vi "Output_Trav_Pos.vi"(4 "Positions to Output":T1) -> (1 "error out":errorcluster)   [LabVIEW 2011]
uses:
  Controls/Positions.ctl
  Globals/Trav_pos_global.vi
  <userlib>/LV-Link3/PolySubVIs/DtCreateAoutChan.vi
  Route mapping/Route_mapping_global.vi
  <userlib>/LV-Link3/PolySubVIs/DtOLWriteSingle.vi
  <userlib>/LV-Link3/PolySubVIs/DtOLWriteMultiple2D.vi
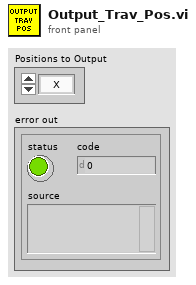
[diagram p1: front panel]
types:
  T1 = typedef "Positions.ctl" = enum16{"X", "Y", "Z", "XY", "XZ", "YZ", "XYZ"}
  T2 = typedef "Box_size.ctl" = cluster{"Max":dbl, "Min":dbl}[]
  T3 = enum32{"Bad", "Idle", "Run top level", "Running"}
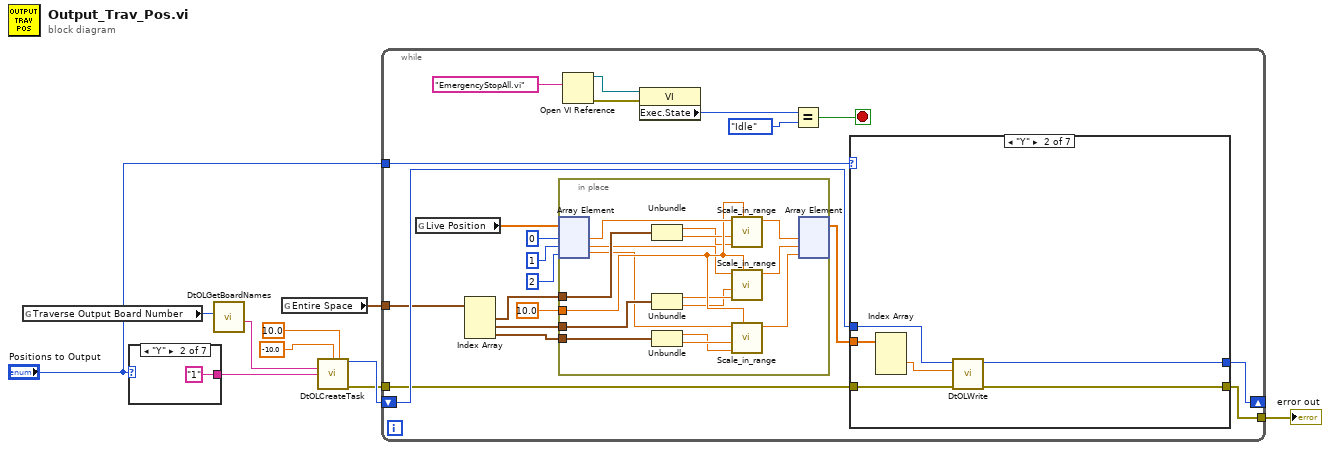
[diagram p0: block diagram]
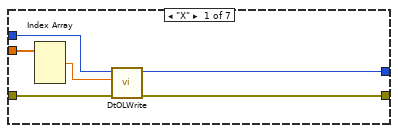
[diagram p2: hidden frame]
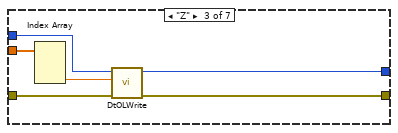
[diagram p3: hidden frame]
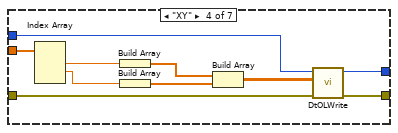
[diagram p4: hidden frame]
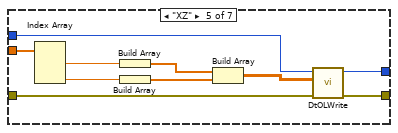
[diagram p5: hidden frame]
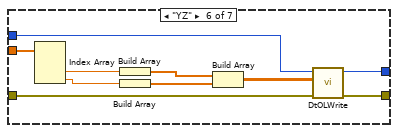
[diagram p6: hidden frame]
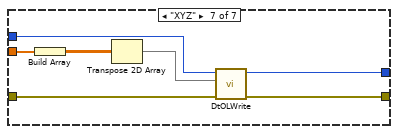
[diagram p7: hidden frame]
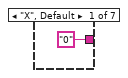
[diagram p8: hidden frame]
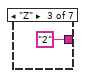
[diagram p9: hidden frame]
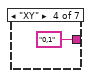
[diagram p10: hidden frame]
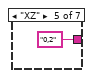
[diagram p11: hidden frame]
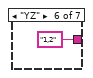
[diagram p12: hidden frame]
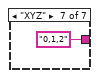
[diagram p13: hidden frame]
diagram:
  n1 = global read "Trav_pos_global.vi" "Traverse Output Board Number"() -> (w2:u32)
  n2 = case shown="\"Y\"" "Positions to Output" {
    tunnel: ["0" ("Channel") "1" ("Channel") "2" ("Channel") "0,1" ("Channel") "0,2" ("Channel") "1,2" ("Channel") "0,1,2" ("Channel")] -> w6
    frame "X", Default {
    }
    frame "Y" {
    }
    frame "Z" {
    }
    frame "XY" {
    }
    frame "XZ" {
    }
    frame "YZ" {
    }
    frame "XYZ" {
    }
  }
  n3 = call <userlib>:"DtOLGetBoardNames.vi"("Select Board"=w2) -> ("Board Name"=w7:string)  [unwired: 8 in, 2 out]
  n4 = global read "Route_mapping_global.vi" "Entire Space"() -> (w1:T2)
  n5 = call-poly <userlib>:"DtOLCreateTask.vi"("Range Min"=-10.0, "Range Max"=10.0, "Board Name"=w7, "Channel"=w6) -> ("Task out"=w8:i32, "error out"=w4:errorcluster)  [unwired: 9 in, 1 out]
  n6 = while {
    shift-right: [w38] -> _
    shift-left: w8 -> [w37]
    tunnel: "Positions to Output" -> [w36]
    tunnel: w4 -> [w29]
    tunnel: [w28] -> w3
    tunnel: w1 -> [w24]
    stop <- w30 stop-if-true
    n7 = global read "Trav_pos_global.vi" "Live Position"() -> (w27:dbl[])
    n8 = Index Array(array=w24) -> (element #1=w23:cluster{"Max":dbl, "Min":dbl}, element #2=w22:cluster{"Max":dbl, "Min":dbl}, element #3=w21:cluster{"Max":dbl, "Min":dbl})  [unwired: 3 in]
    n9 = in-place {
      in-place-border: 10.0 ("Scale Factor") -> [w53]
      in-place-border: w23 -> [w52]
      in-place-border: w22 -> [w49]
      in-place-border: w21 -> [w48]
      n10 = in-place-array #1(w27, 0, 1, 2) -> (w54:dbl, w43:dbl, w42:dbl)
      n11 = Unbundle(w52) -> ("Max"=w50:dbl, "Min"=w51:dbl)
      n12 = Unbundle(w49) -> ("Max"=w45:dbl, "Min"=w44:dbl)
      n13 = Unbundle(w48) -> ("Max"=w46:dbl, "Min"=w47:dbl)
      n14 = call "Scale_in_range.vi"("Scale Factor"=w53, "Maximum Range"=w50, "Minimum Range"=w51, "x"=w54) -> ("Scaled x"=w41:dbl)  [unwired: 7 in]
      n15 = call "Scale_in_range.vi"("Scale Factor"=w53, "Maximum Range"=w45, "Minimum Range"=w44, "x"=w43) -> ("Scaled x"=w40:dbl)  [unwired: 7 in]
      n16 = call "Scale_in_range.vi"("Scale Factor"=w53, "Maximum Range"=w46, "Minimum Range"=w47, "x"=w42) -> ("Scaled x"=w39:dbl)  [unwired: 7 in]
      n17 = in-place-array #1(w41, w40, w39) -> (w26:dbl[])  [unwired: 3 out]
    }
    n18 = Open VI Reference(vi path="EmergencyStopAll.vi") -> (vi reference=w32:refnum<vi>, error out=w33:errorcluster)  [unwired: 5 in]
    n19 = property class="VI"(reference=w32, error in=w33) -> ("Exec.State"=w35:T3)  [unwired: 2 out]
    n20 = Equal?(x=w35, y=T3."Idle") -> (x = y?=w30:bool)
    n21 = case shown="\"Y\"" w36 {
      tunnel: [w60 w66 w72 w82 w92 w102 w107] -> w38
      tunnel: w37 -> [w59 w65 w71 w81 w91 w101 w108]
      tunnel: w26 -> [w57 w63 w70 w80 w90 w100 w109]
      tunnel: w29 -> [w56 w62 w68 w74 w84 w94 w104]
      tunnel: [w55 w61 w67 w73 w83 w93 w103] -> w28
      frame "X" {
        n22 = Index Array(array=w57) -> (element #1=w58:dbl)  [unwired: 3 in, 2 out]
        n23 = call-poly <userlib>:"DtOLWrite.vi"("error in (no error)"=w56, "Data In"=w58, "Task in"=w59) -> ("error out"=w55:errorcluster, "Task out"=w60:i32)  [unwired: 7 in]
      }
      frame "Y" {
        n24 = Index Array(array=w63) -> (element #2=w64:dbl)  [unwired: 3 in, 2 out]
        n25 = call-poly <userlib>:"DtOLWrite.vi"("error in (no error)"=w62, "Data In"=w64, "Task in"=w65) -> ("error out"=w61:errorcluster, "Task out"=w66:i32)  [unwired: 7 in]
      }
      frame "Z" {
        n26 = Index Array(array=w70) -> (element #3=w69:dbl)  [unwired: 3 in, 2 out]
        n27 = call-poly <userlib>:"DtOLWrite.vi"("error in (no error)"=w68, "Data In"=w69, "Task in"=w71) -> ("error out"=w67:errorcluster, "Task out"=w72:i32)  [unwired: 7 in]
      }
      frame "XY" {
        n28 = Index Array(array=w80) -> (element #1=w79:dbl, element #2=w78:dbl)  [unwired: 3 in, 1 out]
        n29 = Build Array(w79) -> (w76:dbl[])
        n30 = Build Array(w78) -> (w77:dbl[])
        n31 = Build Array(w76, w77) -> (w75:dbl[][])
        n32 = call-poly <userlib>:"DtOLWrite.vi"("error in (no error)"=w74, "Data in"=w75, "Task in"=w81) -> ("error out"=w73:errorcluster, "Task out"=w82:i32)  [unwired: 6 in, 1 out]
      }
      frame "XZ" {
        n33 = Index Array(array=w90) -> (element #1=w89:dbl, element #3=w85:dbl)  [unwired: 3 in, 1 out]
        n34 = Build Array(w89) -> (w87:dbl[])
        n35 = Build Array(w85) -> (w88:dbl[])
        n36 = Build Array(w87, w88) -> (w86:dbl[][])
        n37 = call-poly <userlib>:"DtOLWrite.vi"("error in (no error)"=w84, "Data in"=w86, "Task in"=w91) -> ("error out"=w83:errorcluster, "Task out"=w92:i32)  [unwired: 6 in, 1 out]
      }
      frame "YZ" {
        n38 = Index Array(array=w100) -> (element #2=w95:dbl, element #3=w96:dbl)  [unwired: 3 in, 1 out]
        n39 = Build Array(w95) -> (w98:dbl[])
        n40 = Build Array(w96) -> (w99:dbl[])
        n41 = Build Array(w98, w99) -> (w97:dbl[][])
        n42 = call-poly <userlib>:"DtOLWrite.vi"("error in (no error)"=w94, "Data in"=w97, "Task in"=w101) -> ("error out"=w93:errorcluster, "Task out"=w102:i32)  [unwired: 6 in, 1 out]
      }
      frame "XYZ" {
        n43 = Build Array(w109) -> (w106:dbl[][])
        n44 = Transpose 2D Array(2D array=w106) -> (transposed array=w105:dbl[][])
        n45 = call-poly <userlib>:"DtOLWrite.vi"("error in (no error)"=w104, "Data in"=w105, "Task in"=w108) -> ("error out"=w103:errorcluster, "Task out"=w107:i32)  [unwired: 6 in, 1 out]
      }
    }
  }
  "error out" <- w3
